vi "AndorCalculateImageAreaPixelScale.vi"(9 "Y Resolution":i32, 10 "X Resolution":i32, 11 "Image Area:Size:All Elements":cluster{"Width":u32, "Height":u32}) -> (2 "Numeric 2":dbl, 3 "Numeric":dbl)   [LabVIEW 2018, in "AndorOWN.lvlib"]
uses:
  AndorOWN.lvlib
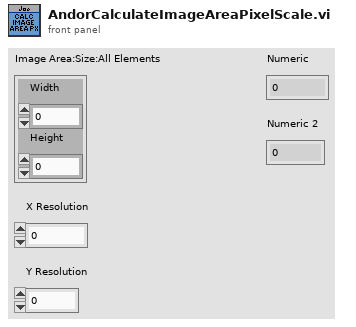
[diagram p1: front panel]
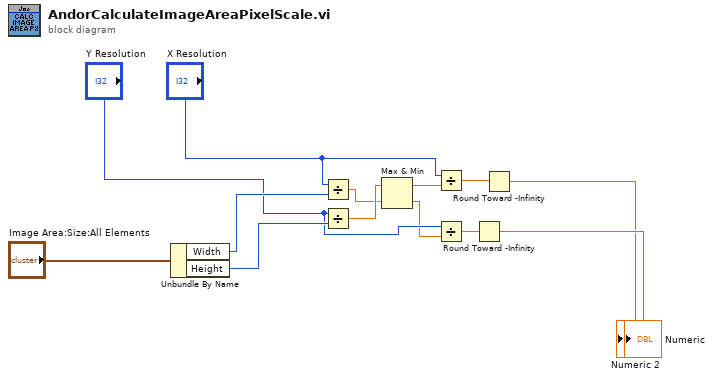
[diagram p0: block diagram]
diagram:
  n1 = Unbundle By Name("Image Area:Size:All Elements") -> ("Width"=w13:u32, "Height"=w12:u32)
  n2 = Divide(x="X Resolution", y=w13) -> (x/y=w1:dbl)
  n3 = Divide(x="Y Resolution", y=w12) -> (x/y=w2:dbl)
  n4 = Max & Min(x=w2, y=w1) -> (max(x,y)=w3:dbl, min(x,y)=w4:dbl)
  n5 = Divide(x="X Resolution", y=w3) -> (x/y=w5:dbl)
  n6 = Divide(x="Y Resolution", y=w4) -> (x/y=w6:dbl)
  n7 = Round Toward -Infinity(1:w6) -> (0:→"Numeric":dbl)
  n8 = Round Toward -Infinity(1:w5) -> (0:→"Numeric 2":dbl)
